vi "From Veristand To Modbus.vi"(7 "Parameters":T1 {"Interface Data"."Serial Settings"."parity (even)" items=["None", "Odd", "Even", "Mark", "Space"]; "Interface Data"."Serial Settings"."flow control (none)" items=["None", "XON/XOFF", "RTS/CTS", "XON/XOFF & RTS/CTS", "DTR/DSR", "XON/XOFF & DTR/DSR"]}, 8 "error in (no error)":errorcluster, 10 "Process in":refnum<class "Process.lvclass">, 11 "Modbus Master in":refnum<class "Modbus Master.lvclass">) -> ()   [LabVIEW 2015, in "Modbus Master Engine.lvlib"]
uses:
  Modbus Master Engine.lvlib
  <vilib>/addons/Inline Async API/_VS Inline Async API/Process/Process.lvclass
  Shared/Device Info.ctl
  Shared/Controls/Interface Type.ctl
  Shared/Controls/Data Model/TCP Settings.ctl
  Shared/Controls/Data Model/Serial Settings.ctl
  Bulk Data Access.ctl
  System Explorer/SubVIs/Modbus Type.ctl
  Shared/Controls/Data Model/Channel.ctl
  <vilib>/NI Veristand/Custom Device API/Custom Device Channel Type.ctl
  Shared/Controls/Data Model/Mapping.ctl
  Shared/Controls/Data Model/DataType.ctl
  <vilib>/NI Veristand/Custom Device API/Custom Device Item Ref.ctl
  Modbus API.lvlibp/API/Master/Modbus Master.lvclass
  <vilib>/addons/Inline Async API/_VS Inline Async API/Process/Process.lvclass/Process.ctl
  <vilib>/addons/Inline Async API/_Data Access Engine/Access Type Classes/Read/Read.lvclass/Read.ctl
  <vilib>/addons/Inline Async API/_Data Access Engine/Data Access Engine/Methods/Read.Data.vi
  <vilib>/addons/Inline Async API/_VS Inline Async API/Process/Data Member Access/Read Data Access.vi
  <vilib>/addons/Inline Async API/_Data Access Engine/Access Type Classes/Read/Read.ProcessData.vi
  <vilib>/addons/Inline Async API/_Data Access Engine/Data Access Engine/Methods/Write.Lookup.vi
  <vilib>/addons/Inline Async API/_Data Access Engine/Data Access Engine/Data Access Engine.lvclass
  Shared/Modbus Master Shared.lvlib
  <vilib>/NI VeriStand/Custom Device API/Custom Device API.lvlib
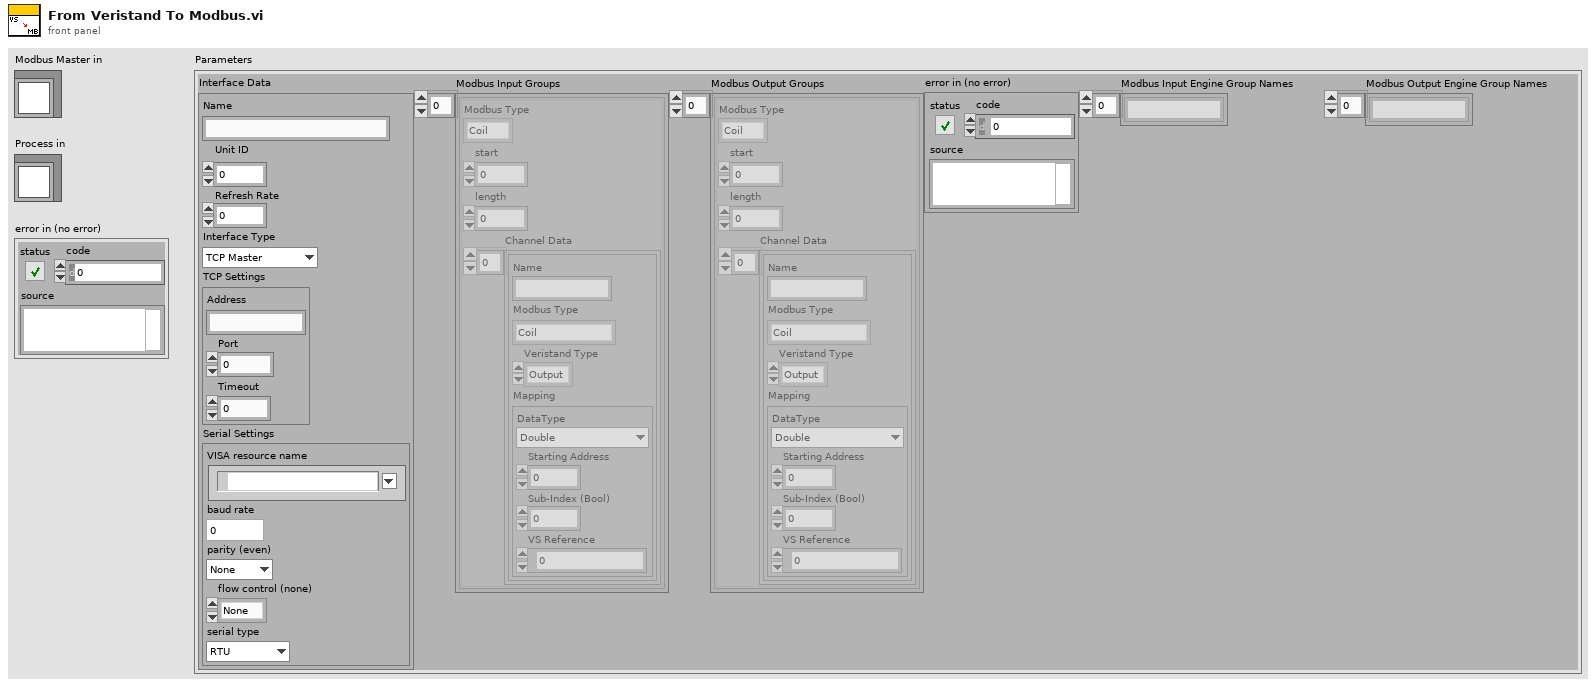
[diagram p1: front panel]
types:
  T1 = typedef "Modbus Master Shared.lvlib/Device Info.ctl" = cluster{"Interface Data":cluster{"Name":string, "Unit ID":u8, "Refresh Rate":i32, "Interface Type":T2, "TCP Settings":T3, "Serial Settings":T4}, "Modbus Input Groups":T5[], "Modbus Output Groups":T5[], "error in (no error)":errorcluster, "Modbus Input Engine Group Names":string[], "Modbus Output Engine Group Names":string[]}
  T2 = typedef "Modbus Master Shared.lvlib/Interface Type.ctl" = enum16{"TCP Master", "Serial Master"}
  T3 = typedef "Modbus Master Shared.lvlib/TCP Settings.ctl" = cluster{"Address":string, "Port":u16, "Timeout":i32}
  T4 = typedef "Modbus Master Shared.lvlib/Serial Settings.ctl" = cluster{"VISA resource name":refnum<visa-resource-name>, "baud rate":u32, "parity (even)":u16, "flow control (none)":u16, "serial type":enum16{"RTU", "ASCII"}}
  T5 = typedef "Modbus Master Shared.lvlib/Bulk Data Access.ctl" = cluster{"Modbus Type":T6, "start":u16, "length":u16, "Channel Data":T7[]}
  T6 = typedef "Modbus Master Shared.lvlib/Modbus Type.ctl" = enum16{"Coil", "Discrete Input", "Holding Register", "Input Register"}
  T7 = typedef "Modbus Master Shared.lvlib/Channel.ctl" = cluster{"Name":string, "Modbus Type":T6, "Veristand Type":T8, "Mapping":T9}
  T8 = typedef "Custom Device API.lvlib/Custom Device Channel Type.ctl" = enum16{"Input", "Output"}
  T9 = typedef "Modbus Master Shared.lvlib/Mapping.ctl" = cluster{"DataType":T10, "Starting Address":u16, "Sub-Index (Bool)":u16, "VS Reference":T11}
  T10 = typedef "Modbus Master Shared.lvlib/DataType.ctl" = enum16{"Double", "Single", "I64", "I32", "I16", "I8", "U64", "U32", "U16", "U8", "Boolean"}
  T11 = typedef "Custom Device API.lvlib/Custom Device Item Ref.ctl" = u64
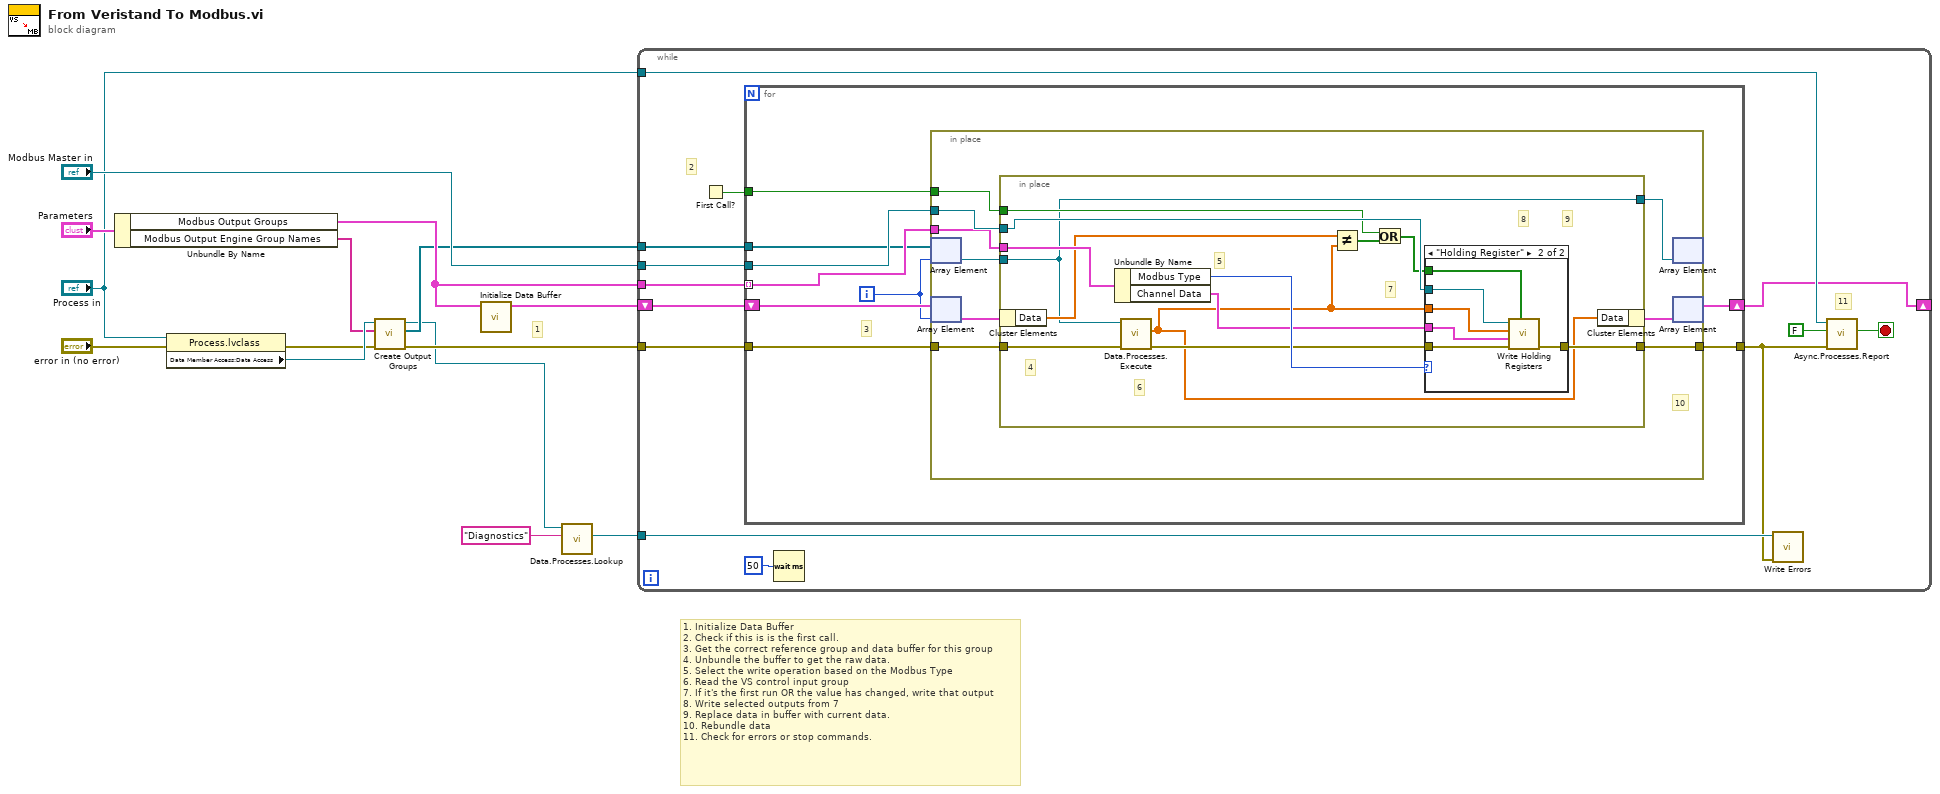
[diagram p0: block diagram]
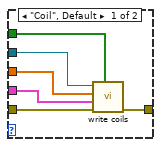
[diagram p2: hidden frame]
diagram:
  # "1"
  # "1. Initialize Data Buffer\n2. Check if this is is the first call.\n3. Get the correct reference group and data buffer for this group\n4. Unbundle the buffer to get the raw data.\n5. Select the write operation based on the Modbus Type\n6. Read the VS control input group\n7. If it's the first run OR the value has changed, write that output\n8. Write selected outputs from 7\n9. Replace data in buffer with current data.\n10. Rebundle data\n11. Check for errors or stop commands."
  n1 = Unbundle By Name("Parameters") -> ("Modbus Output Groups"=w12:T5[], "Modbus Output Engine Group Names"=w8:string[])
  n2 = property class="Process.lvclass"(reference="Process in", error in="error in (no error)") -> (error out=w5:errorcluster, "Data Member Access:Data Access"=w9:refnum<class "Data Access Engine.lvclass">)  [unwired: 1 out]
  n3 = call "Create Output Groups.vi"("error in"=w5, "Input Engine Group Names"=w8, "Data Access Engine in"=w9) -> ("error out"=w4:errorcluster, "Array"=w7:refnum<data-value>[], "Data Access Engine out"=w3:refnum<class "Data Access Engine.lvclass">)  [unwired: 6 in]
  n4 = call "Initialize Data Buffer.vi"("Output Groups"=w12) -> ("Data Buffers"=w11:cluster{"Data":dbl[]}[])  [unwired: 10 in]
  n5 = call-poly <vilib>:"Data.Processes.Lookup.vi"("Name"="Diagnostics", "Data Access API in"=w3) -> ("Ref"=w1:refnum<data-value>)  [unwired: 7 in, 2 out]
  n6 = while {
    tunnel: "Process in" -> [w27]
    tunnel: w7 -> [w24]
    tunnel: w12 -> [w26]
    tunnel: "Modbus Master in" -> [w25]
    tunnel: w4 -> [w23]
    shift-right: [w20] -> _
    shift-left: w11 -> [w21]
    tunnel: w1 -> [w16]
    stop <- w22 stop-if-true
    # "11"
    # "2"
    n7 = First Call?() -> (First Call?: T/F=w17:bool)
    n8 = for {
      tunnel: w26 -> [w35] mode=indexing
      tunnel: w25 -> [w36]
      tunnel: w24 -> [w30]
      tunnel: w23 -> [w34]
      tunnel: [w33] -> w15
      shift-right: [w31] -> w20
      shift-left: w21 -> [w32]
      tunnel: w17 -> [w28]
      i -> [w29]
      # "3"
      n9 = in-place {
        in-place-border: w36 -> [w45]
        in-place-border: w35 -> [w44]
        in-place-border: w34 -> [w43]
        in-place-border: [w42] -> w33
        in-place-border: w28 -> [w37]
        # "10"
        n10 = in-place-array #1(w30, w29) -> (w39:refnum<data-value>)
        n11 = in-place-array #2(w32, w29) -> (w41:cluster{"Data":dbl[]})
        n12 = in-place {
          in-place-border: w45 -> [w58]
          in-place-border: w44 -> [w57]
          in-place-border: w43 -> [w49]
          in-place-border: [w56] -> w42
          in-place-border: w39 -> [w50]
          in-place-border: [w50] -> w38
          in-place-border: w37 -> [w51]
          # "8"
          # "5"
          # "7"
          # "6"
          # "9"
          # "4"
          n13 = in-place-cluster #3(w41) -> ("Data"=w52:dbl[])
          n14 = Unbundle By Name(w57) -> ("Modbus Type"=w55:T6, "Channel Data"=w54:T7[])
          n15 = call-poly <vilib>:"Data.Processes.Execute.vi"("error in (no error)"=w49, "Ref"=w50) -> ("error out"=w48:errorcluster, "Values"=w46:dbl[])  [unwired: 7 in, 1 out]
          n16 = Not Equal?(x=w52, y=w46) -> (x != y?=w53:bool[])
          n17 = Or(x=w51, y=w53) -> (x .or. y?=w47:bool[])
          n18 = case shown="\"Holding Register\"" w55 {
            tunnel: w58 -> [w64 w70]
            tunnel: [w63 w69] -> w56
            tunnel: w48 -> [w62 w68]
            tunnel: w54 -> [w59 w67]
            tunnel: w47 -> [w61 w66]
            tunnel: w46 -> [w60 w65]
            frame "Coil", Default {
              n19 = call "write coils.vi"("Array"=w61, "error in (no error)"=w62, "Channel Data"=w59, "Values"=w60, "Modbus Master in"=w64) -> ("error out"=w63:errorcluster)  [unwired: 6 in]
            }
            frame "Holding Register" {
              n20 = call "Write Holding Registers.vi"("Regs to Write"=w66, "error in (no error)"=w68, "Channel Data"=w67, "Values"=w65, "Modbus Master in"=w70) -> ("error out"=w69:errorcluster)  [unwired: 6 in]
            }
          }
          n21 = in-place-cluster #3("Data"=w46) -> (w40:cluster{"Data":dbl[]})
        }
        n22 = in-place-array #1(w38) -> ()  [unwired: 2 out]
        n23 = in-place-array #2(w40) -> (w31:cluster{"Data":dbl[]}[])  [unwired: 1 out]
      }
    }
    n24 = Wait (ms)(milliseconds to wait=u32 50) -> ()  [unwired: 1 out]
    n25 = call "Write Errors.vi"("error in (no error)"=w15, "Data Value Reference in"=w16) -> ()  [unwired: 10 in]
    n26 = call <vilib>:"Async.Processes.Report.vi"("Error"=w15, "Stop on Error?"=FALSE, "Process in"=w27) -> ("Stop"=w22:bool)  [unwired: 7 in, 1 out]
  }
